vi "reglage-newSD.vi"(0 "How many?":i32=-1) -> (1 "OD":T1(array[cluster]), 2 "SC":T2(array[cluster]))   [LabVIEW 2015]
uses:
  globalVarSD.vi
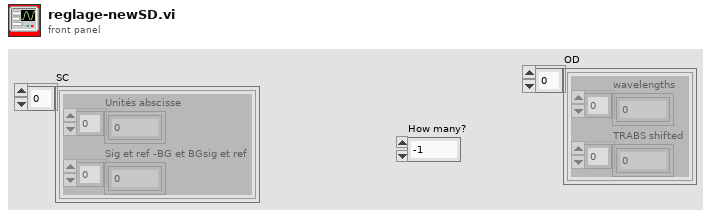
[diagram p1: front panel]
types:
  T1 = cluster{"wavelengths":dbl[], "TRABS shifted":dbl[]}[]
  T2 = cluster{"Unités abscisse":dbl[], "Sig et ref -BG et BGsig et ref":dbl[]}[]
  T3 = typedef "data-cluster.ctl" = cluster{"BG":i32[], "Ie":i32[], "I0":i32[]}[]
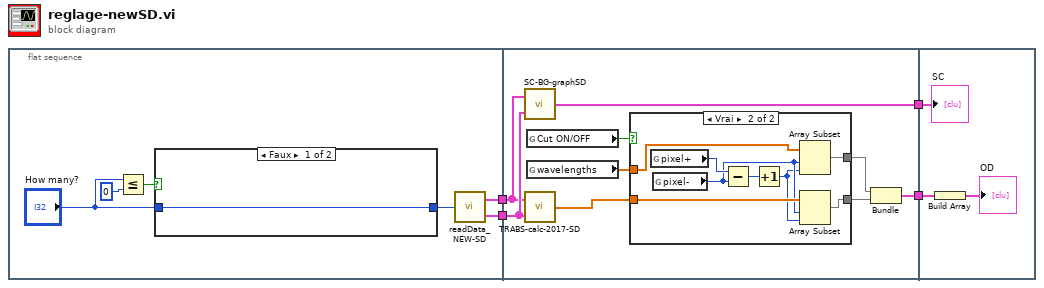
[diagram p0: block diagram]
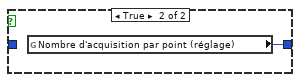
[diagram p2: hidden frame]
diagram:
  n1 = flat-sequence {
    tunnel: [w10] -> w4
    tunnel: [w9] -> w3
    tunnel: w4 -> [w18]
    tunnel: w3 -> [w19]
    tunnel: [w21] -> w2
    tunnel: [w20] -> w1
    tunnel: w2 -> [w33]
    tunnel: w1 -> [w34]
    frame #0 {
      n2 = Less Or Equal?(x="How many?", y=0) -> (x <= y?=w7:bool)
      n3 = case shown="Faux" w7 {
        tunnel: [w11 w12] -> w8
        tunnel: "How many?" -> [w11 _]
        frame False {
        }
        frame True {
          n4 = global read "globalVarSD.vi" "Nombre d'acquisition par point (réglage)"() -> (w12:u32)
        }
      }
      n5 = call "readData_NEW-SD.vi"("number of aq"=w8) -> ("I channel seq"=w10:T3, "II channel seq"=w9:T3)
    }
    frame #1 {
      n6 = call "SC-BG-graphSD.vi"("II channel seq"=w19, "I channel seq"=w18) -> ("Array"=w20:cluster{"wavelengths":dbl[], "Tableau":dbl[]}[])
      n7 = call "TRABS-calc-2017-SD.vi"("II channel seq"=w19, "I channel seq"=w18) -> ("TRABS"=w13:dbl[])
      n8 = global read "globalVarSD.vi" "Cut ON/OFF"() -> (w14:bool)
      n9 = global read "globalVarSD.vi" "wavelengths"() -> (w17:dbl[])
      n10 = case shown="Vrai" w14 {
        tunnel: w17 -> [w23 w31]
        tunnel: [w23 w30] -> w16
        tunnel: w13 -> [w22 w29]
        tunnel: [w22 w28] -> w15
        frame False {
        }
        frame True {
          n11 = global read "globalVarSD.vi" "pixel+"() -> (w26:i32)
          n12 = global read "globalVarSD.vi" "pixel-"() -> (w25:i32)
          n13 = Subtract(x=w26, y=w25) -> (x-y=w27:i32)
          n14 = Increment(x=w27) -> (x+1=w24:i32)
          n15 = Array Subset(array=w31, index=w25, length=w24) -> (w30:dbl[])
          n16 = Array Subset(array=w29, index=w25, length=w24) -> (w28:dbl[])
        }
      }
      n17 = Bundle("wavelengths"=w16, "TRABS"=w15) -> (w21:cluster{"wavelengths":dbl[], "TRABS":dbl[]})  [unwired: 1 in]
    }
    frame #2 {
      n18 = Build Array(w33) -> (→"OD":cluster{"wavelengths":dbl[], "TRABS":dbl[]}[])
      "SC" <- w34
    }
  }
